vi "DriverStationPushData.vi"   [LabVIEW 2019]
doc: "This VI continously sends data from the robot to the FRC 4265 Dashboard, the joysticks, and the FIRST Driver Station. Data are only sent to the network tables when values change. Detailed sensor data are only sent when the user is currently viewing the Tune tab on the FRC 4265 Dashboard."
uses:
  c0b3d222-824d-4eea-b194-4551ccfede72.vi
  63edfc8b-2713-4fb9-bbf0-712b13f7ed91.vi
  47525084-8b38-4927-a12e-3277279b993f.vi
  d8a7f094-08f7-44ee-91a1-5c2b5429b39c.vi
  44ded92d-a7ba-4657-b5b2-ad49251b8caf.vi
  d08dce08-1be1-4dee-a0e2-c808c9915b05.vi
  15eb04b3-c7cc-413a-8ed9-eedb9a2cc229.vi
  681defd6-d800-4e3b-a797-16019fc6eedf.vi
  0e7df65d-03a0-4ac1-9552-43e36140545b.vi
  b779ffbc-e0af-4d3a-a5ff-be904ee9d282.vi
  0fd5d72e-0bbf-454b-88f5-b8f6b912b732.vi
  5dc304d7-e71b-4cd2-8d9d-954937278b50.vi
  d9008cc5-1a39-451b-ae4e-8b2f85e295b1.vi
  d8235c72-9df9-42cd-ba32-07eb0cd93dcc.vi
  bf4cb368-df87-4f8c-8ec5-36368c9759d6.vi
  49b8d36d-15f1-4191-8f66-294e1bcc7d8b.vi
  964589b7-616f-40ea-b924-ce4975bcd482.vi
  ef54d06c-9ef5-4b3b-9535-1c9b0141c808.vi
  a87e27e3-ca91-4abb-bacd-ddf2a2cd984d.vi
  8f6ab1f9-5983-4917-be41-7b146f8af2a0.vi
  e6e35d87-eb7f-4093-a21c-b277472d45f9.vi
  2aaa0aac-34fa-43e5-8230-50058d384c92.vi
  a59d850d-7f58-4d81-8596-951e7b208772.vi
  cbbdf295-aa1d-4db8-8566-cac5820e4458.vi
  cb0926b4-f1bf-44dc-b329-07cb041a7937.vi
  9304f89f-4e24-484b-bf07-7340ed265390.vi
  52d993e2-6fbc-4ee4-b085-b3f80a4c3067.vi
  5ccc8aa6-325d-4660-b060-52e30b1d582a.vi
  296afef1-bc02-48ee-92b6-09523bb21575.vi
  040c557e-2b24-4d13-8fef-d98c711cf45f.vi
  1f68a4f0-bf48-409b-8a47-05a383b8c80c.vi
  68f74b03-6e04-47e5-994a-d14a491b94e1.vi
  811948b9-57e2-4f47-a6f6-f2932d14082f.vi
  14b5543d-6c71-48a0-b45a-be28725dcbfb.vi
  f31b310c-46e7-4cd5-9fe8-a6567badd324.vi
  5739ca73-a30d-4c92-9c50-72d6edc45fc4.vi
  56ff39be-8205-408b-a45a-dea65133fdf1.vi
  fb087c59-fbb1-4979-ba7d-d29f083bcd8a.vi
  0620df73-5841-450f-a219-dd10bb38cbc0.vi
  19ffed08-3a44-4784-ac1f-7d90d09850a5.vi
  95ad0fcc-40ee-4df3-97bc-b677a5e96101.vi
  36759aca-d9c6-44a3-918a-9a0e895c718f.vi
  a94ab05d-8057-462d-9f55-82e7ca490213.vi
  d2dc3f3f-39b5-4c17-a933-05bbedc8d5d9.vi
  47e8091e-0604-4560-b6ee-932fcc40f94c.vi
  9f98788f-6f1b-4a83-a100-7d872b9f460c.vi
  d5b4d43d-cd94-4278-ad04-5030dc28ac17.vi
  89115614-314f-44eb-b4c5-fafba5d31cd4.vi
  04ef483a-e181-4338-9f4a-5a8af9dab594.vi
  2e5da8e6-26da-41d5-8406-8d052fc7da1f.vi
  63edfc8b-2713-4fb9-bbf0-712b13f7ed91.vi/2c9a3d09-8d13-4682-a95d-7c09e00c815b.vi
  47525084-8b38-4927-a12e-3277279b993f.vi/36b3c1b3-fee1-4a8e-95c8-1e3a62b6d3bc.vi
  d8a7f094-08f7-44ee-91a1-5c2b5429b39c.vi/d180070c-83ed-4627-87a2-b1346721cd2d.vi
  44ded92d-a7ba-4657-b5b2-ad49251b8caf.vi/3fcbc4fe-abbd-4266-930b-2c0df1760c3d.vi
  d08dce08-1be1-4dee-a0e2-c808c9915b05.vi/5ffcdf83-7fb4-4319-bf43-93f1f1de344a.vi
  15eb04b3-c7cc-413a-8ed9-eedb9a2cc229.vi/32ed347c-625c-4998-8705-88b75a0bf546.vi
  681defd6-d800-4e3b-a797-16019fc6eedf.vi/d5d94c85-23f5-4806-a2b2-896fc954bd7b.vi
  0e7df65d-03a0-4ac1-9552-43e36140545b.vi/041bd4ac-049c-40bd-b6a5-48b9eda76c97.vi
  b779ffbc-e0af-4d3a-a5ff-be904ee9d282.vi/22be757d-c0b6-4335-bd1f-1f074b992b8d.vi
  0fd5d72e-0bbf-454b-88f5-b8f6b912b732.vi/fae648f3-5525-47b6-a1f7-e741d4808be7.vi
  5dc304d7-e71b-4cd2-8d9d-954937278b50.vi/dcef8a15-4f6d-413a-af1a-301fd53854a9.vi
  d9008cc5-1a39-451b-ae4e-8b2f85e295b1.vi/14c77181-e2cd-4323-b644-178ecfdca62f.vi
  d8235c72-9df9-42cd-ba32-07eb0cd93dcc.vi/50253de8-9ab5-40c4-b2c9-4c5406883f3b.vi
  bf4cb368-df87-4f8c-8ec5-36368c9759d6.vi/eb803bc6-12f5-4fa8-a203-f97f5aa491b4.vi
  49b8d36d-15f1-4191-8f66-294e1bcc7d8b.vi/2d17930b-8628-4552-89ef-34d900995f67.vi
  964589b7-616f-40ea-b924-ce4975bcd482.vi/1d783961-e8dd-4d8c-99e8-31511c884d7c.vi
  ef54d06c-9ef5-4b3b-9535-1c9b0141c808.vi/f2d03ea9-e1b1-4b02-9978-48d30f9e1af1.vi
  a87e27e3-ca91-4abb-bacd-ddf2a2cd984d.vi/0a02d62b-a93c-4e35-89bb-83c2197b1a3e.vi
  8f6ab1f9-5983-4917-be41-7b146f8af2a0.vi/2e926944-275c-41a8-810c-ffebfe3bacc4.vi
  e6e35d87-eb7f-4093-a21c-b277472d45f9.vi/908981bb-5f39-47a4-94fb-cf31480e1e9f.vi
  2aaa0aac-34fa-43e5-8230-50058d384c92.vi/fd494411-181d-4a6d-ae22-44d4baa4a15d.vi
  a59d850d-7f58-4d81-8596-951e7b208772.vi/27a0317e-a8c9-4826-bb51-360108f2f875.vi
  cbbdf295-aa1d-4db8-8566-cac5820e4458.vi/f15bd68e-f182-4cab-8b44-d1c05d7bbdfb.vi
  cb0926b4-f1bf-44dc-b329-07cb041a7937.vi/d4aa75bc-6e2b-46c3-8c7a-4474c43c8772.vi
  9304f89f-4e24-484b-bf07-7340ed265390.vi/909f1667-625f-43da-938f-d58b35225210.vi
  52d993e2-6fbc-4ee4-b085-b3f80a4c3067.vi/0034a970-136e-4ad7-aff3-5ebd95c99a67.vi
  5ccc8aa6-325d-4660-b060-52e30b1d582a.vi/4d9f1b7f-6fed-4279-9a56-4adce5db3ff8.vi
  296afef1-bc02-48ee-92b6-09523bb21575.vi/6232eeb1-ad40-45ba-9019-59370ed63cfe.vi
  040c557e-2b24-4d13-8fef-d98c711cf45f.vi/c9d06e64-4af8-4166-b414-96a318fa7fcf.vi
  1f68a4f0-bf48-409b-8a47-05a383b8c80c.vi/e3993fce-27c4-47a7-a405-d9a45bab0c6f.vi
  68f74b03-6e04-47e5-994a-d14a491b94e1.vi/28362545-a9fe-44fc-b083-bdc58be5256e.vi
  811948b9-57e2-4f47-a6f6-f2932d14082f.vi/dbe29640-659d-4489-9c98-f9c4abcbd9e2.vi
  14b5543d-6c71-48a0-b45a-be28725dcbfb.vi/c59ab7a4-af08-4ebc-90a6-c1bf8d064b8a.vi
  f31b310c-46e7-4cd5-9fe8-a6567badd324.vi/45c0bdab-316f-46a2-9a76-71224d80f76b.vi
  5739ca73-a30d-4c92-9c50-72d6edc45fc4.vi/946ceb12-d64b-4c88-b330-efb7316e520d.vi
  56ff39be-8205-408b-a45a-dea65133fdf1.vi/eed03e83-566d-4792-bea4-764e1f848191.vi
  fb087c59-fbb1-4979-ba7d-d29f083bcd8a.vi/66808fe3-61ef-41a6-b9a9-f57b0a28a3db.vi
  0620df73-5841-450f-a219-dd10bb38cbc0.vi/19ecee36-c2a4-47a1-b5ca-6645a047c93d.vi
  19ffed08-3a44-4784-ac1f-7d90d09850a5.vi/2ff6438d-ab4a-40be-8230-af6e6b8cce35.vi
  95ad0fcc-40ee-4df3-97bc-b677a5e96101.vi/2e07175e-482f-4e75-b878-4755de482572.vi
  36759aca-d9c6-44a3-918a-9a0e895c718f.vi/a2c3eec6-eea1-4dd6-86bf-4b919e0b4aee.vi
  a94ab05d-8057-462d-9f55-82e7ca490213.vi/db4f4a7e-5f7d-44e3-8322-cbd1db550af4.vi
  d2dc3f3f-39b5-4c17-a933-05bbedc8d5d9.vi/dc009efe-6848-48dc-af0b-8b9342473125.vi
  47e8091e-0604-4560-b6ee-932fcc40f94c.vi/ef34300c-eaf8-4a9f-ac82-98f873737d86.vi
  9f98788f-6f1b-4a83-a100-7d872b9f460c.vi/836a0433-7627-43e2-bcdd-2f31d936866a.vi
  d5b4d43d-cd94-4278-ad04-5030dc28ac17.vi/5c4daa42-6b61-4c8e-8c44-85e726def382.vi
  89115614-314f-44eb-b4c5-fafba5d31cd4.vi/96514fc7-79b2-4e34-bc32-2d8a2329d594.vi
  04ef483a-e181-4338-9f4a-5a8af9dab594.vi/41f42718-b95f-417b-95e4-024466a04eff.vi
  2e5da8e6-26da-41d5-8406-8d052fc7da1f.vi/f6317036-af06-4075-ad96-f3ab0a76f396.vi
  dsdata.vi
  <vilib>/Rock Robotics/Network Tables/NT Write String.vi
  constants.vi
  <vilib>/Rock Robotics/Network Tables/NT Write String Array.vi
  <vilib>/Rock Robotics/Network Tables/NT Write Number.vi
  sensors.vi
  outputs.vi
  <vilib>/Rock Robotics/Network Tables/NT Write Boolean Array.vi
  <vilib>/Rock Robotics/Network Tables/NT Write Boolean.vi
  autoninfo.vi
  refnums.vi
  GRNF_Joystick.vi
  dsinstructions.vi
types:
  T1 = enum16{"Driver Control", "Auto Targeting", "Feeder Station"}
  T2 = typedef "WPI_DriverStationRobotMode2.ctl" = enum16{"Autonomous Disabled", "Autonomous Enabled", "Teleop Disabled", "Teleop Enabled", "Disconnected", "Finish", "Test Disabled", "Test Enabled", "Emergency Stopped"}
  T3 = typedef "WPI_DriverStationAllianceInfo.ctl" = enum16{"Red", "Blue", "Invalid"}
  T4 = typedef "WPI_JoystickDevRef.ctl" = cluster{"Device":T5}
  T5 = typedef "WPI_JoystickDeviceEnum.ctl" = enum16{"USB 0", "USB 1", "USB 2", "USB 3", "USB 4", "USB 5"}
  T6 = enum16{"Low Gear", "High Gear", "Transiting", "Unknown", "Force Low Gear"}
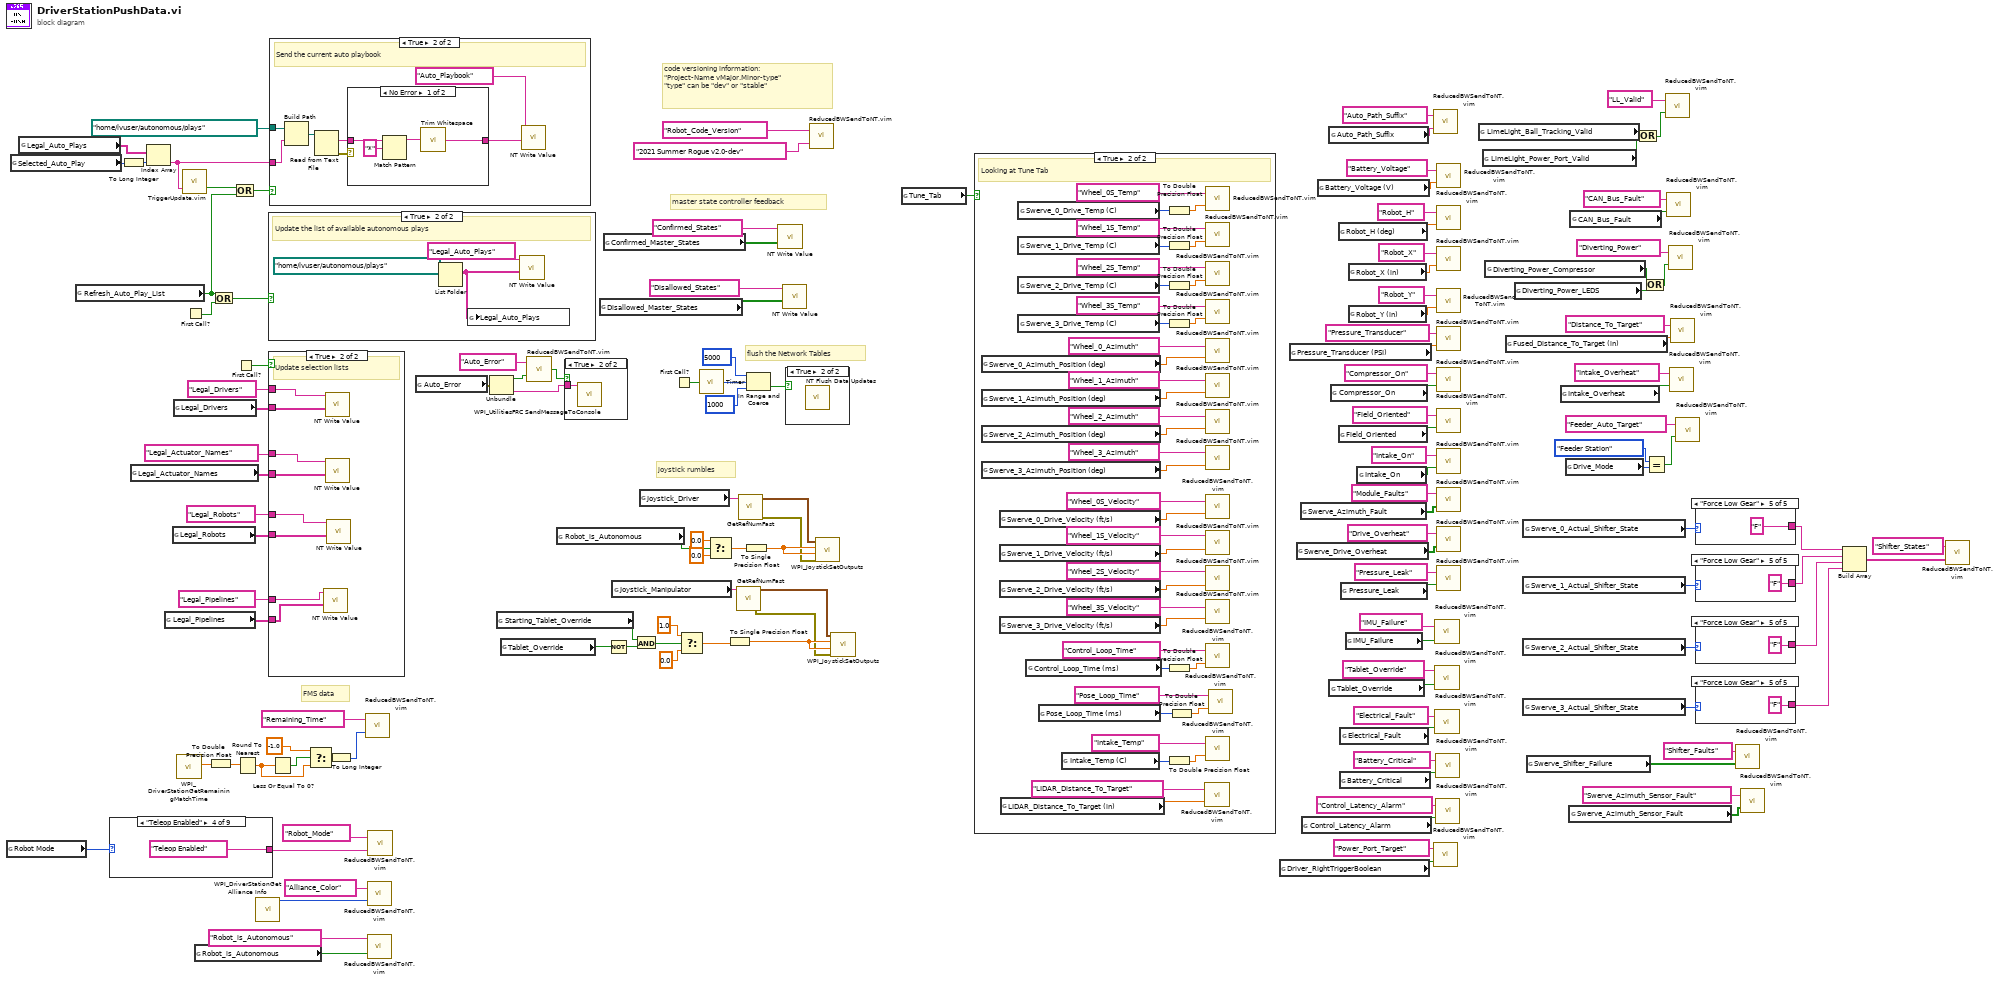
[diagram p0: block diagram]
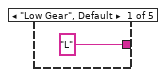
[diagram p3: hidden frame]
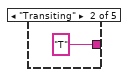
[diagram p4: hidden frame]
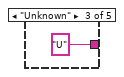
[diagram p5: hidden frame]
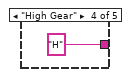
[diagram p6: hidden frame]
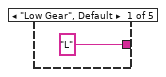
[diagram p7: hidden frame]
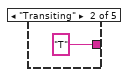
[diagram p8: hidden frame]
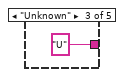
[diagram p9: hidden frame]
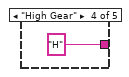
[diagram p10: hidden frame]
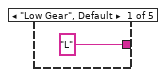
[diagram p11: hidden frame]
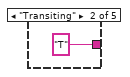
[diagram p12: hidden frame]
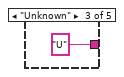
[diagram p13: hidden frame]
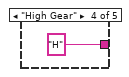
[diagram p14: hidden frame]
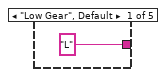
[diagram p15: hidden frame]
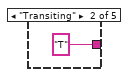
[diagram p16: hidden frame]
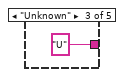
[diagram p17: hidden frame]
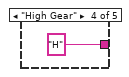
[diagram p18: hidden frame]
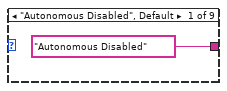
[diagram p19: hidden frame]
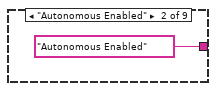
[diagram p20: hidden frame]
diagram:
  # "flush the Network Tables"
  # "code versioning information:\n\"Project-Name vMajor.Minor-type\"\n\"type\" can be \"dev\" or \"stable\""
  # "FMS data"
  # "master state controller feedback"
  # "joystick rumbles"
  n1 = global read "dsdata.vi" "Robot Mode"() -> (w48:T2)
  n2 = global read "dsdata.vi" "Selected_Auto_Play"() -> (w59:u16)
  n3 = global read "constants.vi" "Legal_Auto_Plays"() -> (w60:string[])
  n4 = global read "dsdata.vi" "Refresh_Auto_Play_List"() -> (w39:bool)
  n5 = case shown="\"Teleop Enabled\"" w48 {
    tunnel: ["Autonomous Disabled" "Autonomous Enabled" "Teleop Disabled" "Teleop Enabled" "Disconnected" "Finish" "Test Disabled" "Test Enabled" "Emergency Stopped"] -> w47
    frame "Autonomous Disabled", Default {
    }
    frame "Autonomous Enabled" {
    }
    frame "Teleop Disabled" {
    }
    frame "Teleop Enabled" {
    }
    frame "Disconnected" {
    }
    frame "Finish" {
    }
    frame "Test Disabled" {
    }
    frame "Test Enabled" {
    }
    frame "Emergency Stopped" {
    }
  }
  n6 = To Long Integer(number=w59) -> (32bit integer=w61:i32)
  n7 = global read "constants.vi" "Legal_Actuator_Names"() -> (w70:string[])
  n8 = Index Array(array=w60, index=w61) -> (element=w58:string)
  n9 = global read "constants.vi" "Legal_Pipelines"() -> (w10:string[])
  n10 = global read "constants.vi" "Legal_Robots"() -> (w37:string[])
  n11 = global read "constants.vi" "Legal_Drivers"() -> (w136:string[])
  n12 = call <vilib>:"WPI_DriverStationGetRemainingMatchTime.vi"() -> ("Match Time(s)"=w129:sgl)  [unwired: 10 in, 1 out]
  n13 = call "TriggerUpdate.vim"("Trigger"=w58) -> ("Update"=w41:bool)  [unwired: 2 in]
  n14 = First Call?() -> (First Call?: T/F=w138:bool)
  n15 = global read "dsdata.vi" "Robot_is_Autonomous"() -> (w46:bool)
  n16 = To Double Precision Float(number=w129) -> (double precision float=w133:dbl)
  n17 = Or(x=w39, y=w138) -> (x .or. y?=w137:bool)
  n18 = Or(x=w41, y=w39) -> (x .or. y?=w40:bool)
  n19 = First Call?() -> (First Call?: T/F=w134:bool)
  n20 = Round To Nearest(number=w133) -> (nearest integer value=w50:dbl)
  n21 = call <vilib>:"WPI_DriverStationGet Alliance Info.vi"() -> ("Alliance"=w108:T3)  [unwired: 6 in, 5 out]
  n22 = case shown="True" w137 {
    frame False {
    }
    frame True {
      # "Update the list of available autonomous plays"
      n23 = List Folder(path=path "/home/lvuser/autonomous/plays") -> (filenames=w148:string[])  [unwired: 3 in, 3 out]
      n24 = global write "constants.vi" "Legal_Auto_Plays"(w148) -> ()
      n25 = call-poly <vilib>:"NT Write Value.vi"("String Array"=w148, "Name"="Legal_Auto_Plays") -> ()  [unwired: 9 in, 1 out]
    }
  }
  n26 = case shown="True" w134 {
    tunnel: w136 -> [_ w158]
    tunnel: "Legal_Drivers" ("Name") -> [_ w157]
    tunnel: w70 -> [_ w156]
    tunnel: "Legal_Actuator_Names" ("Name") -> [_ w155]
    tunnel: "Legal_Robots" ("Name") -> [_ w154]
    tunnel: w37 -> [_ w153]
    tunnel: "Legal_Pipelines" ("Name") -> [_ w152]
    tunnel: w10 -> [_ w151]
    frame False {
    }
    frame True {
      # "Update selection lists"
      n27 = call-poly <vilib>:"NT Write Value.vi"("String Array"=w151, "Name"=w152) -> ()  [unwired: 9 in, 1 out]
      n28 = call-poly <vilib>:"NT Write Value.vi"("String Array"=w158, "Name"=w157) -> ()  [unwired: 9 in, 1 out]
      n29 = call-poly <vilib>:"NT Write Value.vi"("String Array"=w156, "Name"=w155) -> ()  [unwired: 9 in, 1 out]
      n30 = call-poly <vilib>:"NT Write Value.vi"("String Array"=w153, "Name"=w154) -> ()  [unwired: 9 in, 1 out]
    }
  }
  n31 = case shown="True" w40 {
    tunnel: path "/home/lvuser/autonomous/plays" ("path") -> [_ w165]
    tunnel: w58 -> [_ w161]
    frame False {
    }
    frame True {
      # "Send the current auto playbook"
      n32 = Build Path(base path=w165, name or relative path=w161) -> (appended path=w164:path)
      n33 = Read from Text File(file (use dialog)=w164) -> (text=w162:string, error out=w163:errorcluster)  [unwired: 3 in, 2 out]
      n34 = case shown="No Error" w163 {
        tunnel: w162 -> [w169 _]
        tunnel: [w168 "Error: No playbook found"] -> w160
        frame No Error {
          n35 = Match Pattern(string=w169, regular expression="*") -> (before substring=w166:string)  [unwired: 1 in, 3 out]
          n36 = call <vilib>:"Trim Whitespace.vi"("string"=w166) -> ("trimmed string"=w168:string)  [unwired: 1 in]
        }
        frame Error {
        }
      }
      n37 = call-poly <vilib>:"NT Write Value.vi"("String"=w160, "Name"="Auto_Playbook") -> ()  [unwired: 9 in, 1 out]
    }
  }
  n38 = Less Or Equal To 0?(x=w50) -> (x <= 0?=w132:bool)
  n39 = Select(t=-1.0, s=w132, f=w50) -> (s? t:f=w131:dbl)
  n40 = To Long Integer(number=w131) -> (32bit integer=w111:i32)
  n41 = call "ReducedBWSendToNT.vim"("Value In"=w111, "NT Name"="Remaining_Time" ("Name")) -> ()  [unwired: 1 out]
  n42 = call "ReducedBWSendToNT.vim"("Value In"=w108, "NT Name"="Alliance_Color" ("Name")) -> ()  [unwired: 1 out]
  n43 = call "ReducedBWSendToNT.vim"("Value In"=w46, "NT Name"="Robot_is_Autonomous") -> ()  [unwired: 1 out]
  n44 = call "ReducedBWSendToNT.vim"("Value In"=w47, "NT Name"="Robot_Mode") -> ()  [unwired: 1 out]
  n45 = global read "autoninfo.vi" "Auto_Error"() -> (w124:errorcluster)
  n46 = Unbundle(w124) -> ("status"=w84:bool, "source"=w123:string)  [unwired: 1 out]
  n47 = global read "dsdata.vi" "Starting_Tablet_Override"() -> (w115:bool)
  n48 = global read "dsdata.vi" "Tablet_Override"() -> (w116:bool)
  n49 = call "ReducedBWSendToNT.vim"("Value In"=w84, "NT Name"="Auto_Error" ("Name")) -> ("Value Changed"=w83:bool)
  n50 = global read "dsdata.vi" "Robot_is_Autonomous"() -> (w44:bool)
  n51 = case shown="True" w83 {
    tunnel: w123 -> [_ w171]
    frame False {
    }
    frame True {
      n52 = call <vilib>:"WPI_UtilitiesFRC SendMessageToConsole.vi"("Message"=w171) -> ()  [unwired: 14 in, 1 out]
    }
  }
  n53 = global read "outputs.vi" "Disallowed_Master_States"() -> (w51:bool[])
  n54 = global read "outputs.vi" "Confirmed_Master_States"() -> (w126:bool[])
  n55 = Not(x=w116) -> (.not. x?=w117:bool)
  n56 = global read "refnums.vi" "Joystick_Manipulator"() -> (w63:string)
  n57 = And(x=w115, y=w117) -> (x .and. y?=w114:bool)
  n58 = global read "refnums.vi" "Joystick_Driver"() -> (w66:string)
  n59 = First Call?() -> (First Call?: T/F=w5:bool)
  n60 = Select(t=1.0, s=w114, f=0.0) -> (s? t:f=w119:dbl)
  n61 = call "Timer.vi"("Reset Timer"=w5) -> ("Time (ms)"=w4:u32)
  n62 = Select(t=0.0, s=w44, f=0.0) -> (s? t:f=w43:dbl)
  n63 = To Single Precision Float(number=w119) -> (single precision float=w118:sgl)
  n64 = call-poly "GetRefNumFast.vi"("RefNum Name"=w63) -> ("Error"=w65:errorcluster, "Device Reference"=w64:T4)  [unwired: 5 in]
  n65 = call-poly "GetRefNumFast.vi"("RefNum Name"=w66) -> ("Error"=w67:errorcluster, "Device Reference"=w68:T4)  [unwired: 5 in]
  n66 = To Single Precision Float(number=w43) -> (single precision float=w122:sgl)
  n67 = In Range and Coerce(upper limit=u32 5000, x=w4, lower limit=u32 1000) -> (In Range?=w1:bool)  [unwired: 1 out]
  n68 = call-poly <vilib>:"NT Write Value.vi"("Boolean Array"=w126, "Name"="Confirmed_States") -> ()  [unwired: 9 in, 1 out]
  n69 = call-poly <vilib>:"NT Write Value.vi"("Boolean Array"=w51, "Name"="Disallowed_States") -> ()  [unwired: 9 in, 1 out]
  n70 = case shown="True" w1 {
    frame False {
    }
    frame True {
      n71 = call <vilib>:"NT Flush Data Updates.vi"() -> ()  [unwired: 11 in, 1 out]
    }
  }
  n72 = call "ReducedBWSendToNT.vim"("Value In"="2021 Summer Rogue v2.0-dev", "NT Name"="Robot_Code_Version" ("Name")) -> ()  [unwired: 1 out]
  n73 = call <vilib>:"WPI_JoystickSetOutputs.vi"("error in (no error)"=w67, "Right Rumble"=w122, "Left Rumble"=w122, "JoystickDevRef"=w68) -> ()  [unwired: 6 in, 2 out]
  n74 = call <vilib>:"WPI_JoystickSetOutputs.vi"("error in (no error)"=w65, "Right Rumble"=w118, "Left Rumble"=w118, "JoystickDevRef"=w64) -> ()  [unwired: 6 in, 2 out]
  n75 = global read "dsdata.vi" "Tune_Tab"() -> (w128:bool)
  n76 = case shown="True" w128 {
    frame False {
      # "Not Looking at Tune Tab"
    }
    frame True {
      # "Looking at Tune Tab"
      n77 = global read "sensors.vi" "Swerve_0_Azimuth_Position (deg)"() -> (w195:dbl)
      n78 = global read "sensors.vi" "Swerve_1_Azimuth_Position (deg)"() -> (w193:dbl)
      n79 = global read "sensors.vi" "Swerve_2_Azimuth_Position (deg)"() -> (w191:dbl)
      n80 = global read "sensors.vi" "Swerve_3_Azimuth_Position (deg)"() -> (w189:dbl)
      n81 = global read "sensors.vi" "Swerve_0_Drive_Velocity (ft/s)"() -> (w187:dbl)
      n82 = global read "sensors.vi" "Swerve_1_Drive_Velocity (ft/s)"() -> (w185:dbl)
      n83 = global read "sensors.vi" "Swerve_2_Drive_Velocity (ft/s)"() -> (w183:dbl)
      n84 = global read "sensors.vi" "Swerve_3_Drive_Velocity (ft/s)"() -> (w181:dbl)
      n85 = global read "sensors.vi" "LIDAR_Distance_To_Target (in)"() -> (w176:dbl)
      n86 = global read "sensors.vi" "Swerve_0_Drive_Temp (C)"() -> (w210:u8)
      n87 = global read "sensors.vi" "Swerve_1_Drive_Temp (C)"() -> (w208:u8)
      n88 = global read "sensors.vi" "Swerve_2_Drive_Temp (C)"() -> (w207:u8)
      n89 = global read "sensors.vi" "Swerve_3_Drive_Temp (C)"() -> (w206:u8)
      n90 = global read "sensors.vi" "Control_Loop_Time (ms)"() -> (w209:u32)
      n91 = global read "sensors.vi" "Pose_Loop_Time (ms)"() -> (w174:u32)
      n92 = global read "sensors.vi" "Intake_Temp (C)"() -> (w205:u8)
      n93 = To Double Precision Float(number=w210) -> (double precision float=w203:dbl)
      n94 = To Double Precision Float(number=w208) -> (double precision float=w201:dbl)
      n95 = To Double Precision Float(number=w207) -> (double precision float=w199:dbl)
      n96 = To Double Precision Float(number=w206) -> (double precision float=w197:dbl)
      n97 = To Double Precision Float(number=w209) -> (double precision float=w179:dbl)
      n98 = To Double Precision Float(number=w205) -> (double precision float=w177:dbl)
      n99 = To Double Precision Float(number=w174) -> (double precision float=w172:dbl)
      n100 = call "ReducedBWSendToNT.vim"("Value In"=w176, "NT Name"="LIDAR_Distance_To_Target") -> ()  [unwired: 1 out]
      n101 = call "ReducedBWSendToNT.vim"("Value In"=w203, "NT Name"="Wheel_0S_Temp" ("Name")) -> ()  [unwired: 1 out]
      n102 = call "ReducedBWSendToNT.vim"("Value In"=w201, "NT Name"="Wheel_1S_Temp" ("Name")) -> ()  [unwired: 1 out]
      n103 = call "ReducedBWSendToNT.vim"("Value In"=w199, "NT Name"="Wheel_2S_Temp" ("Name")) -> ()  [unwired: 1 out]
      n104 = call "ReducedBWSendToNT.vim"("Value In"=w197, "NT Name"="Wheel_3S_Temp" ("Name")) -> ()  [unwired: 1 out]
      n105 = call "ReducedBWSendToNT.vim"("Value In"=w195, "NT Name"="Wheel_0_Azimuth" ("Name")) -> ()  [unwired: 1 out]
      n106 = call "ReducedBWSendToNT.vim"("Value In"=w193, "NT Name"="Wheel_1_Azimuth" ("Name")) -> ()  [unwired: 1 out]
      n107 = call "ReducedBWSendToNT.vim"("Value In"=w191, "NT Name"="Wheel_2_Azimuth" ("Name")) -> ()  [unwired: 1 out]
      n108 = call "ReducedBWSendToNT.vim"("Value In"=w189, "NT Name"="Wheel_3_Azimuth" ("Name")) -> ()  [unwired: 1 out]
      n109 = call "ReducedBWSendToNT.vim"("Value In"=w187, "NT Name"="Wheel_0S_Velocity" ("Name")) -> ()  [unwired: 1 out]
      n110 = call "ReducedBWSendToNT.vim"("Value In"=w185, "NT Name"="Wheel_1S_Velocity" ("Name")) -> ()  [unwired: 1 out]
      n111 = call "ReducedBWSendToNT.vim"("Value In"=w183, "NT Name"="Wheel_2S_Velocity" ("Name")) -> ()  [unwired: 1 out]
      n112 = call "ReducedBWSendToNT.vim"("Value In"=w181, "NT Name"="Wheel_3S_Velocity" ("Name")) -> ()  [unwired: 1 out]
      n113 = call "ReducedBWSendToNT.vim"("Value In"=w179, "NT Name"="Control_Loop_Time" ("Name")) -> ()  [unwired: 1 out]
      n114 = call "ReducedBWSendToNT.vim"("Value In"=w177, "NT Name"="Intake_Temp" ("Name")) -> ()  [unwired: 1 out]
      n115 = call "ReducedBWSendToNT.vim"("Value In"=w172, "NT Name"="Pose_Loop_Time" ("Name")) -> ()  [unwired: 1 out]
    }
  }
  n116 = global read "dsinstructions.vi" "Driver_RightTriggerBoolean"() -> (w8:bool)
  n117 = global read "sensors.vi" "Pressure_Transducer (PSI)"() -> (w98:dbl)
  n118 = global read "sensors.vi" "Swerve_Drive_Overheat"() -> (w88:bool[])
  n119 = global read "sensors.vi" "Swerve_Azimuth_Fault"() -> (w90:bool[])
  n120 = global read "sensors.vi" "Control_Latency_Alarm"() -> (w52:bool)
  n121 = global read "sensors.vi" "Battery_Voltage (V)"() -> (w106:dbl)
  n122 = global read "autoninfo.vi" "Auto_Path_Suffix"() -> (w12:string)
  n123 = global read "dsdata.vi" "Tablet_Override"() -> (w74:bool)
  n124 = global read "sensors.vi" "Compressor_On"() -> (w96:bool)
  n125 = global read "sensors.vi" "Robot_H (deg)"() -> (w104:dbl)
  n126 = global read "outputs.vi" "Field_Oriented"() -> (w94:bool)
  n127 = global read "sensors.vi" "Battery_Critical"() -> (w54:bool)
  n128 = global read "sensors.vi" "Electrical_Fault"() -> (w56:bool)
  n129 = global read "sensors.vi" "Pressure_Leak"() -> (w86:bool)
  n130 = global read "sensors.vi" "IMU_Failure"() -> (w76:bool)
  n131 = global read "sensors.vi" "Robot_X (in)"() -> (w102:dbl)
  n132 = global read "sensors.vi" "Robot_Y (in)"() -> (w100:dbl)
  n133 = global read "outputs.vi" "Intake_On"() -> (w92:bool)
  n134 = call "ReducedBWSendToNT.vim"("Value In"=w12, "NT Name"="Auto_Path_Suffix" ("Name")) -> ()  [unwired: 1 out]
  n135 = call "ReducedBWSendToNT.vim"("Value In"=w8, "NT Name"="Power_Port_Target" ("Name")) -> ()  [unwired: 1 out]
  n136 = call "ReducedBWSendToNT.vim"("Value In"=w76, "NT Name"="IMU_Failure" ("Name")) -> ()  [unwired: 1 out]
  n137 = call "ReducedBWSendToNT.vim"("Value In"=w74, "NT Name"="Tablet_Override" ("Name")) -> ()  [unwired: 1 out]
  n138 = call "ReducedBWSendToNT.vim"("Value In"=w56, "NT Name"="Electrical_Fault" ("Name")) -> ()  [unwired: 1 out]
  n139 = call "ReducedBWSendToNT.vim"("Value In"=w54, "NT Name"="Battery_Critical" ("Name")) -> ()  [unwired: 1 out]
  n140 = call "ReducedBWSendToNT.vim"("Value In"=w52, "NT Name"="Control_Latency_Alarm" ("Name")) -> ()  [unwired: 1 out]
  n141 = call "ReducedBWSendToNT.vim"("Value In"=w106, "NT Name"="Battery_Voltage" ("Name")) -> ()  [unwired: 1 out]
  n142 = call "ReducedBWSendToNT.vim"("Value In"=w104, "NT Name"="Robot_H" ("Name")) -> ()  [unwired: 1 out]
  n143 = call "ReducedBWSendToNT.vim"("Value In"=w102, "NT Name"="Robot_X" ("Name")) -> ()  [unwired: 1 out]
  n144 = call "ReducedBWSendToNT.vim"("Value In"=w100, "NT Name"="Robot_Y" ("Name")) -> ()  [unwired: 1 out]
  n145 = call "ReducedBWSendToNT.vim"("Value In"=w98, "NT Name"="Pressure_Transducer" ("Name")) -> ()  [unwired: 1 out]
  n146 = call "ReducedBWSendToNT.vim"("Value In"=w96, "NT Name"="Compressor_On" ("Name")) -> ()  [unwired: 1 out]
  n147 = call "ReducedBWSendToNT.vim"("Value In"=w94, "NT Name"="Field_Oriented" ("Name")) -> ()  [unwired: 1 out]
  n148 = call "ReducedBWSendToNT.vim"("Value In"=w92, "NT Name"="Intake_On" ("Name")) -> ()  [unwired: 1 out]
  n149 = call "ReducedBWSendToNT.vim"("Value In"=w90, "NT Name"="Module_Faults" ("Name")) -> ()  [unwired: 1 out]
  n150 = call "ReducedBWSendToNT.vim"("Value In"=w88, "NT Name"="Drive_Overheat" ("Name")) -> ()  [unwired: 1 out]
  n151 = call "ReducedBWSendToNT.vim"("Value In"=w86, "NT Name"="Pressure_Leak" ("Name")) -> ()  [unwired: 1 out]
  n152 = global read "sensors.vi" "LimeLight_Ball_Tracking_Valid"() -> (w16:bool)
  n153 = global read "sensors.vi" "LimeLight_Power_Port_Valid"() -> (w15:bool)
  n154 = global read "outputs.vi" "Diverting_Power_Compressor"() -> (w35:bool)
  n155 = global read "sensors.vi" "Fused_Distance_To_Target (in)"() -> (w80:dbl)
  n156 = global read "outputs.vi" "Diverting_Power_LEDS"() -> (w34:bool)
  n157 = global read "sensors.vi" "Swerve_0_Actual_Shifter_State"() -> (w28:T6)
  n158 = global read "sensors.vi" "Swerve_1_Actual_Shifter_State"() -> (w27:T6)
  n159 = global read "sensors.vi" "Swerve_2_Actual_Shifter_State"() -> (w26:T6)
  n160 = global read "sensors.vi" "Swerve_3_Actual_Shifter_State"() -> (w25:T6)
  n161 = global read "sensors.vi" "Swerve_Shifter_Failure"() -> (w18:bool[])
  n162 = global read "sensors.vi" "Intake_Overheat"() -> (w78:bool)
  n163 = global read "outputs.vi" "Drive_Mode"() -> (w113:T1)
  n164 = global read "sensors.vi" "Swerve_Azimuth_Sensor_Fault"() -> (w6:bool[])
  n165 = global read "sensors.vi" "CAN_Bus_Fault"() -> (w32:bool)
  n166 = Or(x=w16, y=w15) -> (x .or. y?=w14:bool)
  n167 = Or(x=w35, y=w34) -> (x .or. y?=w36:bool)
  n168 = Equal?(x=T1."Feeder Station", y=w113) -> (x = y?=w72:bool)
  n169 = call "ReducedBWSendToNT.vim"("Value In"=w14, "NT Name"="LL_Valid" ("Name")) -> ()  [unwired: 1 out]
  n170 = call "ReducedBWSendToNT.vim"("Value In"=w32, "NT Name"="CAN_Bus_Fault" ("Name")) -> ()  [unwired: 1 out]
  n171 = call "ReducedBWSendToNT.vim"("Value In"=w36, "NT Name"="Diverting_Power" ("Name")) -> ()  [unwired: 1 out]
  n172 = call "ReducedBWSendToNT.vim"("Value In"=w78, "NT Name"="Intake_Overheat" ("Name")) -> ()  [unwired: 1 out]
  n173 = call "ReducedBWSendToNT.vim"("Value In"=w80, "NT Name"="Distance_To_Target" ("Name")) -> ()  [unwired: 1 out]
  n174 = call "ReducedBWSendToNT.vim"("Value In"=w72, "NT Name"="Feeder_Auto_Target" ("Name")) -> ()  [unwired: 1 out]
  n175 = case shown="\"Force Low Gear\"" w28 {
    tunnel: ["L" "T" "U" "H" "F"] -> w24
    frame "Low Gear", Default {
    }
    frame "Transiting" {
    }
    frame "Unknown" {
    }
    frame "High Gear" {
    }
    frame "Force Low Gear" {
    }
  }
  n176 = case shown="\"Force Low Gear\"" w27 {
    tunnel: ["L" "T" "U" "H" "F"] -> w23
    frame "Low Gear", Default {
    }
    frame "Transiting" {
    }
    frame "Unknown" {
    }
    frame "High Gear" {
    }
    frame "Force Low Gear" {
    }
  }
  n177 = case shown="\"Force Low Gear\"" w26 {
    tunnel: ["L" "T" "U" "H" "F"] -> w22
    frame "Low Gear", Default {
    }
    frame "Transiting" {
    }
    frame "Unknown" {
    }
    frame "High Gear" {
    }
    frame "Force Low Gear" {
    }
  }
  n178 = case shown="\"Force Low Gear\"" w25 {
    tunnel: ["L" "T" "U" "H" "F"] -> w21
    frame "Low Gear", Default {
    }
    frame "Transiting" {
    }
    frame "Unknown" {
    }
    frame "High Gear" {
    }
    frame "Force Low Gear" {
    }
  }
  n179 = call "ReducedBWSendToNT.vim"("Value In"=w18, "NT Name"="Shifter_Faults") -> ()  [unwired: 1 out]
  n180 = call "ReducedBWSendToNT.vim"("Value In"=w6, "NT Name"="Swerve_Azimuth_Sensor_Fault" ("Name")) -> ()  [unwired: 1 out]
  n181 = Build Array(w24, w23, w22, w21) -> (w20:string[])
  n182 = call "ReducedBWSendToNT.vim"("Value In"=w20, "NT Name"="Shifter_States") -> ()  [unwired: 1 out]
